vi "__List Drives.vi"(8 "error in (no error)":errorcluster) -> (0 "error out":errorcluster, 2 "Drive letters":string[](array[string]), 3 "Drive paths":path[](array[path]))   [LabVIEW 2011]
doc: "Return the list of drive letters and their associated paths found on the local computer."
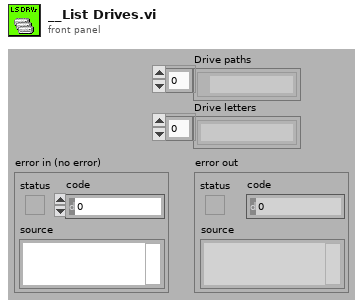
[diagram p1: front panel]
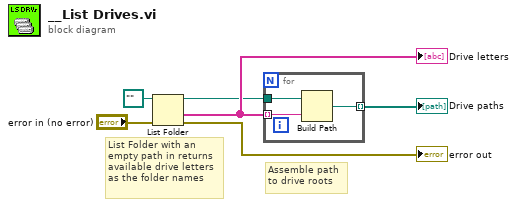
[diagram p0: block diagram]
diagram:
  # "Assemble path\nto drive roots"
  # "List Folder with an\nempty path in returns\navailable drive letters\nas the folder names"
  n1 = List Folder(path=path "", error in="error in (no error)") -> (path out=w2:path, folder names=w3:string[], error out=→"error out":errorcluster)  [unwired: 2 in, 1 out]
  "Drive letters" <- w3
  n2 = for {
    tunnel: w3 -> [w9] mode=indexing
    tunnel: w2 -> [w8]
    tunnel: [w7] -> w1 mode=indexing
    n3 = Build Path(base path=w8, name or relative path=w9) -> (appended path=w7:path)
  }
  "Drive paths" <- w1
